vi "Get Subscriptions.vi"(8 "error in (no error)":errorcluster, 11 "Test Double Data Tracker in":refnum<class "Test Double Data Tracker.lvclass">) -> (0 "error out":errorcluster, 2 "Subscriptions":refnum<class "Data.lvclass">[](array[class]), 3 "Test Double Data Tracker out":refnum<class "Test Double Data Tracker.lvclass">)   [LabVIEW 2020, in "Test.lvlib" / "Test Double Data Tracker.lvclass"]
doc: "Return the subscriptions associated with the instance of the Data Tracker Msg."
uses:
  Test Double Data Tracker.lvclass
  PPL/HDH.Data.Generic.lvlibp/Data.lvclass
  Data/Test Double Data/Test Double Data.lvclass
  C:/Current projects/WS/PPL/HDH.Data.Generic.lvlibp/Data.lvclass
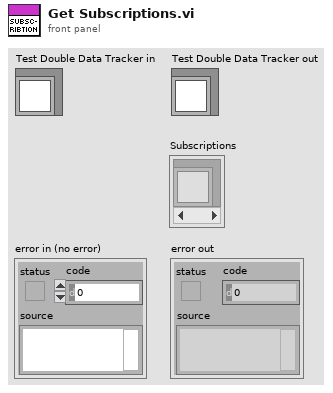
[diagram p1: front panel]
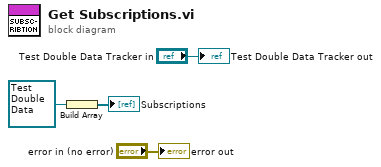
[diagram p0: block diagram]
diagram:
  n1 = Build Array(refnum<class "Test Double Data.lvclass"> refnum ("Test.lvlib:Test Double Data.lvclass")) -> (→"Subscriptions":refnum<class "Test Double Data.lvclass">[])
  "error out" <- "error in (no error)"
  "Test Double Data Tracker out" <- "Test Double Data Tracker in"
